vi "RDS Child Receive Message.vi"(8 "error in (no error)":errorcluster, 10 "RDS Message":refnum<class "RDS Message.lvclass">, 11 "RDS Controller Actor in":refnum<class "RDS Controller Actor.lvclass">) -> (0 "error out":errorcluster, 3 "RDS Controller Actor out":refnum<class "RDS Controller Actor.lvclass">)   [LabVIEW 2015, in "RDS Controller Actor.lvlib" / "RDS Controller Actor.lvclass"]
uses:
  RDS Controller Actor.lvclass
  Libraries/RDS Framework/RDS Message Class/RDS Message.lvclass
  Libraries/RDS Framework/RDS Message Class/RDS Message.lvclass/RDS Message.ctl
  Libraries/RDS Child Messages/Controller Message/Controller Message.lvclass
  Libraries/RDS Child Messages/Controller Message/Controller Message.lvclass/Controller Message.ctl
  <vilib>/ActorFramework/Actor/Actor.lvclass/Actor.ctl
  <vilib>/ActorFramework/Message Enqueuer/Message Enqueuer.lvclass/Message Enqueuer.ctl
  <vilib>/ActorFramework/Message Enqueuer/Init from Existing Queue.vi
  <vilib>/ActorFramework/Message Enqueuer/Message Enqueuer.lvclass
  RDS Controller Actor Messages/Controller Send State Msg/Controller Send State Msg.lvclass
  <vilib>/ActorFramework/Actor/Actor.lvclass
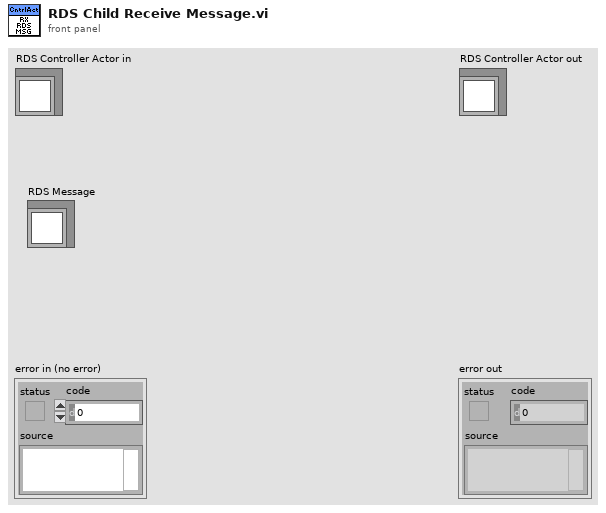
[diagram p1: front panel]
types:
  T1 = typedef "RDS Child Messages.lvlib/RDS Message ID.ctl" = enum16{"RDS Hello World", "String Message", "AIP_Status", "AIP_Command", "GPS_Data", "MCB_Command", "MCB_Status", "Compass_Data", "Depth_Data", "Battery_Data", "Contoller_State", "Set_Mag_Dev", "BTB_Shutdown", "State_Sample_Request", "State_Sample", "PID_Gains_Set", "Helm_Limiter_Set", "Helm_Heading_Command", "Helm_Steering_Command", "Helm_Status", "Controller_Message", "AIP_Set_Min_Depth", "Mission_Controller_State", "Mission_Upload", "Mission_Set_Op_and_Run", "Mission_Settings_Set"}
  T2 = typedef "RDS Controller Actor.lvlib/Controller.ctl" = enum16{"Idle", "Local Remote Control", "Shore Remote Control", "Mission Control"}
  T3 = typedef "RDS Child Messages.lvlib/Controller Message.lvclass/Controller Message Type.ctl" = enum16{"Control Relinquish Request", "Control Relinquish Command", "Control Request", "Control Granted"}
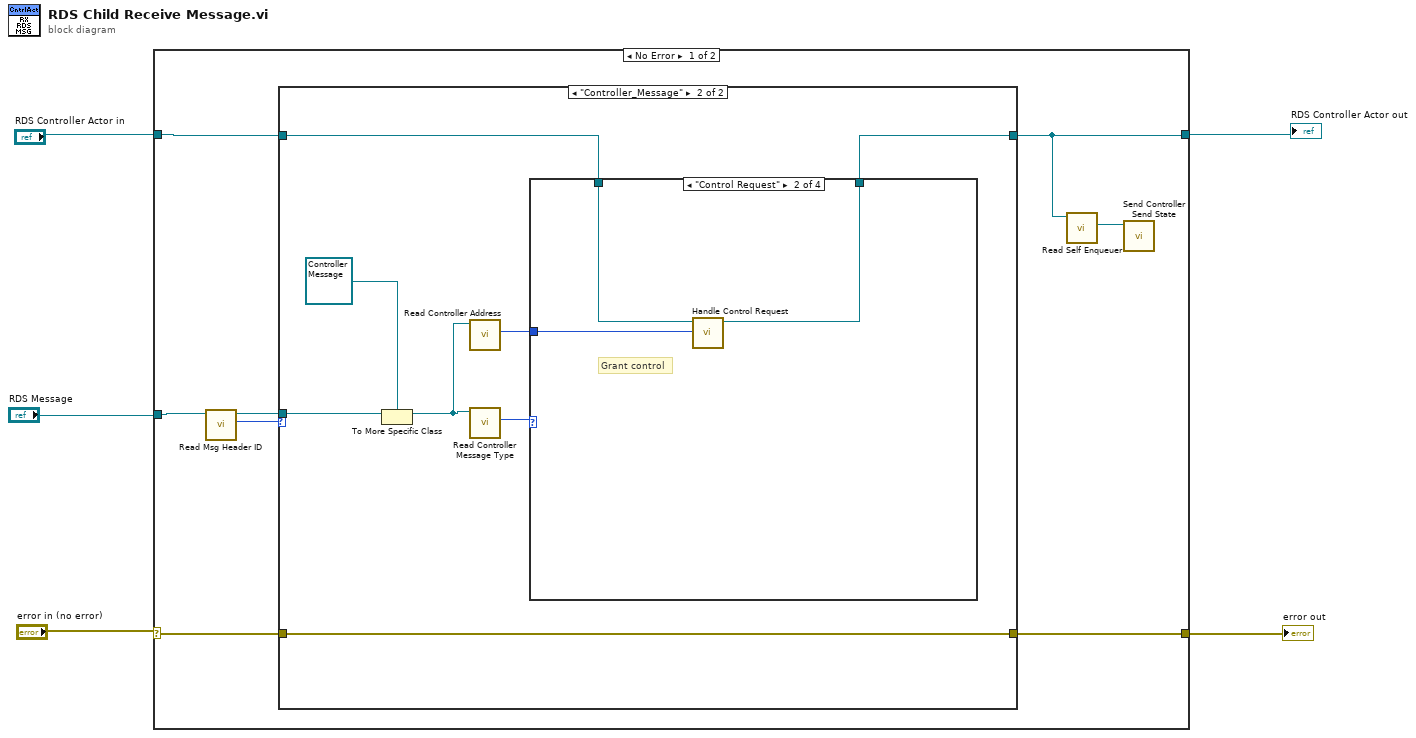
[diagram p0: block diagram]
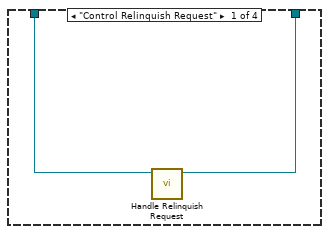
[diagram p3: hidden frame]
diagram:
  n1 = case shown="No Error" "error in (no error)" {
    selector: "error in (no error)" -> [w9 w31]
    tunnel: "RDS Message" -> [w13 _]
    tunnel: "RDS Controller Actor in" -> [w8 w32]
    tunnel: [w7 w32] -> w4
    tunnel: [w10 w31] -> w1
    frame No Error {
      n2 = call "Read Msg Header ID.vi"("RDS Message in"=w13) -> ("Msg ID"=w12:T1, "RDS Message out"=w11:refnum<class "RDS Message.lvclass">)  [unwired: 6 in, 3 out]
      n3 = case shown="\"Controller_Message\"" w12 {
        tunnel: w11 -> [_ w23]
        tunnel: [w15 w22] -> w10
        tunnel: w9 -> [w15 w22]
        tunnel: w8 -> [w14 w18]
        tunnel: [w14 w17] -> w7
        frame "RDS Hello World", Default {
        }
        frame "Controller_Message" {
          n4 = To More Specific Class(target class=refnum<class "Controller Message.lvclass"> refnum ("RDS Child Messages.lvlib:Controller Message.lvclass"), reference=w23) -> (specific class reference=w20:refnum<class "Controller Message.lvclass">)  [unwired: 1 in, 1 out]
          n5 = call "Read Controller Address.vi"("Controller Message in"=w20) -> ("Controller"=w16:T2)  [unwired: 8 in, 2 out]
          n6 = call "Read Controller Message Type.vi"("Controller Message in"=w20) -> ("Controller Message Type"=w19:T3)  [unwired: 8 in, 2 out]
          n7 = case shown="\"Control Request\"" w19 {
            tunnel: w18 -> [w25 w27 w29 w30]
            tunnel: [w24 w26 w29 w30] -> w17
            tunnel: w16 -> [_ w28 _ _]
            frame "Control Relinquish Request" {
              n8 = call "Handle Relinquish Request.vi"("RDS Controller Actor in"=w25) -> ("RDS Controller Actor out"=w24:refnum<class "RDS Controller Actor.lvclass">)  [unwired: 9 in, 1 out]
            }
            frame "Control Request" {
              # "Grant control"
              n9 = call "Handle Control Request.vi"("Command Requester"=w28, "RDS Controller Actor in"=w27) -> ("RDS Controller Actor out"=w26:refnum<class "RDS Controller Actor.lvclass">)  [unwired: 8 in, 1 out]
            }
            frame "Control Granted" {
              # "This message insn't for us"
            }
            frame "Control Relinquish Command" {
              # "This message insn't for us"
            }
          }
        }
      }
      n10 = call <vilib>:"Read Self Enqueuer.vi"("Actor"=w7) -> ("Self Enqueuer"=w6:refnum<class "Message Enqueuer.lvclass">)  [unwired: 10 in]
      n11 = call "Send Controller Send State.vi"("Message Enqueuer in"=w6) -> ()  [unwired: 9 in, 2 out]
    }
    frame Error {
    }
  }
  "error out" <- w1
  "RDS Controller Actor out" <- w4
